vi "FTW-Supervisor-Connect.vi"(5 "Supervisor Address":string, 11 "error in":errorcluster) -> (4 "FTW Supervisor Connection":refnum<class "FTW-Supervisor-Connector.lvclass">, 15 "error out":errorcluster)   [LabVIEW 2014, in "FTW-Supervisor-Connector.lvclass"]
uses:
  FTW-Supervisor-Connector.lvclass
  connector/FTW-Actor-Connector.lvclass
panel:
  # "Inputs"
  # "Outputs"
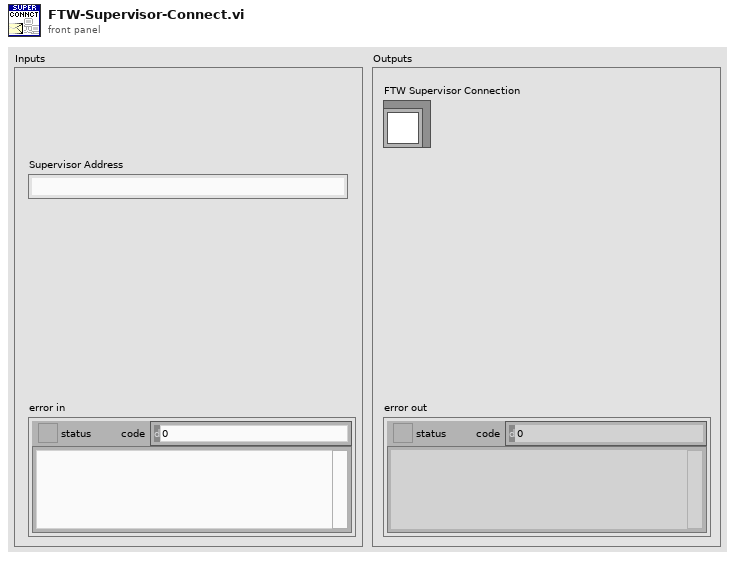
[diagram p1: front panel]
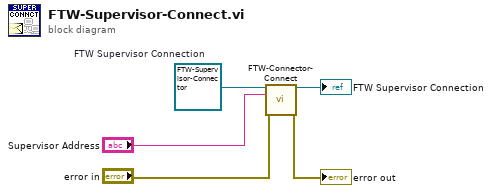
[diagram p0: block diagram]
diagram:
  w2 = refnum<class "FTW-Supervisor-Connector.lvclass"> refnum  # FTW Supervisor Connection
  n1 = call "FTW-Connector-Connect.vi"("FTW Actor Connector"=w2, "Instance Inbox Address"="Supervisor Address", "error in"="error in") -> ("FTW Actor Connector out"=→"FTW Supervisor Connection":refnum<class "FTW-Supervisor-Connector.lvclass">, "error out"=→"error out":errorcluster)  [unwired: 11 in]
